vi "Read Graph-Chart Plot Names.vi"(8 "error in":errorcluster, 11 "Graph / Chart Reference in":refnum<vi>) -> (0 "error out":errorcluster, 1 "Value":string[](array[string]), 2 "Interpret As Unicode":bool, 3 "Graph / Chart Reference out":refnum<vi>)   [LabVIEW 2020, in "G-Unicode.lvlib"]
uses:
  Unicode/SubVIs/Byte Order Marks.vi
  G-Unicode.lvlib
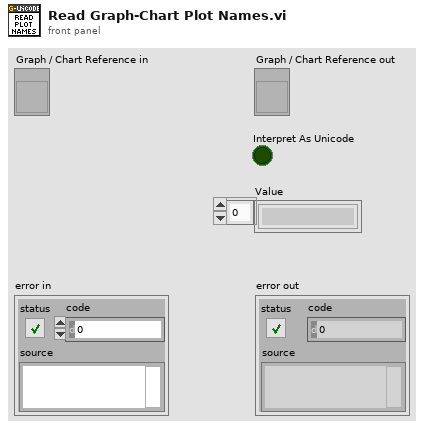
[diagram p1: front panel]
types:
  T1 = typedef "LVCursorListTypeDef.ctl" = cluster{"Name":string, "Color":u32, "Style":u8, "Point Style":u8, "Name Visible":bool, "Allow Drag":bool, "Cursor Mode":u32, "Plot":i32, "Index":i32, "Position":cluster{"X":dbl, "Y":dbl}, "X Scale":u32, "Y Scale":u32, "Watch Plots":i32[], "Watch All Plots":bool, "Plot Area":i32, "Label Offset":cluster{"X":dbl, "Y":dbl}}[]
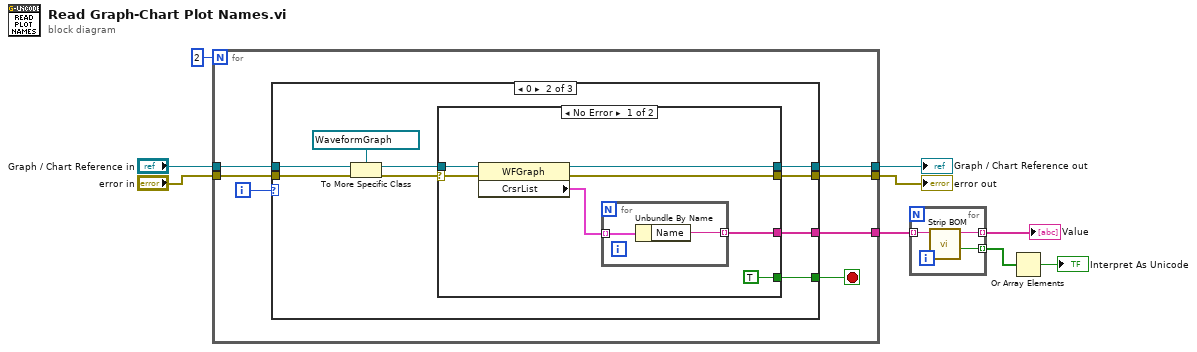
[diagram p0: block diagram]
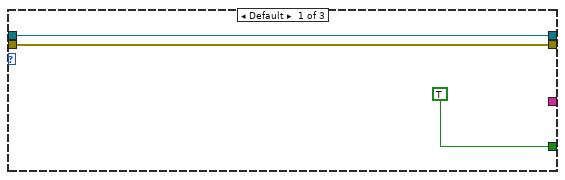
[diagram p2: hidden frame]
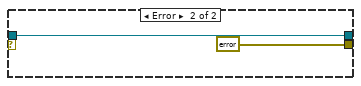
[diagram p3: hidden frame]
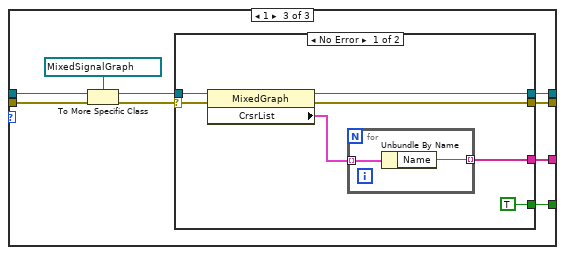
[diagram p4: hidden frame]
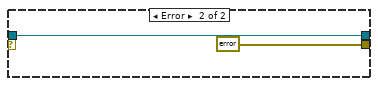
[diagram p5: hidden frame]
diagram:
  n1 = for {
    N: 2 -> [_]
    tunnel: "error in" -> [w16]
    tunnel: [w15] -> w8
    tunnel: [w14] -> w7
    tunnel: "Graph / Chart Reference in" -> [w13]
    tunnel: [w10] -> w3
    i -> [w12]
    stop <- w11 stop-if-true
    n2 = case shown="0" w12 {
      tunnel: w16 -> [w18 w24 w44]
      tunnel: [w19 w28 w48] -> w15
      tunnel: [w18 w27 w47] -> w14
      tunnel: w13 -> [w19 w26 w46]
      tunnel: [TRUE w21 w41] -> w11
      tunnel: [_ w20 w40] -> w10
      frame Default {
      }
      frame 0 {
        n3 = To More Specific Class(target class=refnum<vi> refnum ("Graph / Chart Reference in"), reference=w26, error in=w24) -> (specific class reference=w25:refnum<vi>, error out=w22:errorcluster)
        n4 = case shown="No Error" w22 {
          selector: w22 -> [w32 _]
          tunnel: [w35 w38] -> w28
          tunnel: [w34 errorcluster {"status"=FALSE, "code"=0, "source"=""} ("error IO")] -> w27
          tunnel: w25 -> [w33 w38]
          tunnel: [TRUE _] -> w21
          tunnel: [w29 _] -> w20
          frame No Error {
            n5 = property class="WFGraph"(reference=w33, error in=w32) -> (reference out=w35:refnum<vi>, error out=w34:errorcluster, "CrsrList"=w30:T1)
            n6 = for {
              tunnel: w30 -> [w37] mode=indexing
              tunnel: [w36] -> w29 mode=indexing
              n7 = Unbundle By Name(w37) -> ("Name"=w36:string)
            }
          }
          frame Error {
          }
        }
      }
      frame 1 {
        n8 = To More Specific Class(target class=refnum<vi> refnum ("Graph / Chart Reference in"), reference=w46, error in=w44) -> (specific class reference=w45:refnum<vi>, error out=w42:errorcluster)
        n9 = case shown="No Error" w42 {
          selector: w42 -> [w52 _]
          tunnel: [w55 w58] -> w48
          tunnel: [w54 errorcluster {"status"=FALSE, "code"=0, "source"=""} ("error IO")] -> w47
          tunnel: w45 -> [w53 w58]
          tunnel: [TRUE _] -> w41
          tunnel: [w49 _] -> w40
          frame No Error {
            n10 = property class="MixedGraph"(reference=w53, error in=w52) -> (reference out=w55:refnum<vi>, error out=w54:errorcluster, "CrsrList"=w50:T1)
            n11 = for {
              tunnel: w50 -> [w57] mode=indexing
              tunnel: [w56] -> w49 mode=indexing
              n12 = Unbundle By Name(w57) -> ("Name"=w56:string)
            }
          }
          frame Error {
          }
        }
      }
    }
  }
  "error out" <- w7
  "Graph / Chart Reference out" <- w8
  n13 = for {
    tunnel: w3 -> [w62] mode=indexing
    tunnel: [w61] -> w2 mode=indexing
    tunnel: [w60] -> w4 mode=indexing
    n14 = call "Strip BOM.vi"("String"=w62) -> ("BOM Found"=w60:bool, "String without BOM"=w61:string)  [unwired: 8 in, 1 out]
  }
  "Value" <- w2
  n15 = Or Array Elements(Boolean array=w4) -> (logical OR=→"Interpret As Unicode":bool)
